vi "MasterAquisitionFile_FP.vi"() -> ()   [LabVIEW 2020]
uses:
  <vilib>/userDefined/High Color/IMAQdx.ctl
  <vilib>/vision/driver/IMAQdx.llb/IMAQdx Camera Control Mode.ctl
  <vilib>/vision/driver/IMAQdx.llb/IMAQdx Acquisition Mode.ctl
  <vilib>/vision/driver/IMAQdx.llb/IMAQdx Buffer Number Mode.ctl
  <vilib>/DAQmx/write.llb/DAQmx Write (Digital 1D Wfm NChan NSamp).vi
  <vilib>/DAQmx/read.llb/DAQmx Read (Digital 1D Bool 1Chan 1Samp).vi
  <vilib>/DAQmx/read.llb/DAQmx Read (Analog 1D Wfm NChan NSamp).vi
  <vilib>/Waveform/DWDTOps.llb/DWDT Digital to Boolean Array.vi
  <vilib>/DAQmx/create/channels.llb/DAQmx Create Channel (DO-Digital Output).vi
  <vilib>/DAQmx/configure/timing.llb/DAQmx Timing (Sample Clock).vi
  <vilib>/Waveform/DWDTOps.llb/DWDT Boolean Array to Digital.vi
  <vilib>/Waveform/DWDTOps.llb/DWDT Uncompress Digital.vi
  <vilib>/DAQmx/miscellaneous.llb/DAQmx Fill In Error Info.vi
  <vilib>/DAQmx/create/channels.llb/DAQmx Create Channel (DI-Digital Input).vi
  <vilib>/DAQmx/create/channels.llb/DAQmx Create Channel (AI-Voltage-Basic).vi
  <vilib>/DAQmx/configure/trigger.llb/DAQmx Start Trigger (Digital Edge).vi
  <vilib>/DAQmx/create/channels.llb/DAQmx Create Channel (CO-Pulse Generation-Frequency).vi
  <vilib>/DAQmx/configure/timing.llb/DAQmx Timing (Implicit).vi
  <vilib>/vision/driver/NI_Vision_Acquisition_Software.lvlib
  <resource>/objmgr/imaqdx.rc
  <resource>/objmgr/daqmx.rc
panel:
  in  "Analog Input Channels":tag="Dev2/ai0:3"
  out "Auditory":bool
  out "RPad":bool
  out "LPad":bool
  in  "Sol Stim Parameters":cluster{"Fs":dbl, "Samples":dbl}
  in  "LED Stim Parameters":cluster{"Fs":dbl, "Samples":dbl}
  in  "Generate Stimuli":bool=TRUE
  in  "Sol Duty Cycle (%)":dbl=50.0
  in  "Sol Freq":dbl=5.0
  in  "Sol Dur (s)":dbl=5.0
  in  "LED Duty Cycle (%)":dbl=10.0
  in  "LED Freq":dbl=10.0
  in  "LED Dur (s)":dbl=2.0
  out "Stimulus Order":digitalwaveform[](graph)=[{"t0"=timestamp(0 s since 1904-01-01), "dt"=5e-05, "Y"={"transitions"=[], "data"=array19221000x1[19221000 elements]}}, {"t0"=timestamp(0 s since 1904-01-01), "dt"=5e-05, "Y"={"transitions"=[], "data"=array19221000x1[19221000 elements]}}, {"t0"=timestamp(0 s since 1904-01-01), "dt"=5e-05, "Y"={"transitions"=[], "data"=array19221000x1[19221000 elements]}}]
  out "Solenoid Stim":digitalwaveform(graph)={"t0"=timestamp(0 s since 1904-01-01), "dt"=5e-05, "Y"={"transitions"=[], "data"=array100000x1[100000 elements]}}
  in  "Trial Offset (s)":dbl=45.0
  in  "Interstim (s)":dbl=45.0
  in  "Right Pad":dbl=1.0
  in  "Left Pad":dbl=1.0
  in  "Auditory":dbl=1.0
  in  "LED":dbl
  out "?":T1(plugin-control)
  in  "stop":bool
  out "?":T1(plugin-control)
  out "Behavior Cam Fs":dbl(knob) scale=0.0..200.0
  out "Behav Cam":bool
  out "Complete":bool
  out "Whisk Cam":bool
  out "Analog":bool
  out "MScan Trig":bool
  out "?":bool[](array[boolean])=[TRUE]
  out "Hexadecimal Data":u32=1 format="%x"
  out "Time Elapsed (Min)":cluster{dbl, dbl}(slide)={16.0, 0.0} scale=0.0..16.0 scale format="%#_2g"
  out "Whisker Camera":bool
  out "Analog Data":bool
  out "Analog Samples":i32=15417328
  in  "Device Analog Channel Labels":string[](array[string])=["forceSensor", "LPadSol", "RPadSol", "AudSol", "", "", "", ""]
  in  "?":cluster{"Analog Fs":u16}={"Analog Fs"=20000} {"Analog Fs" format="%0.0f"}
  in  "?":cluster{"WhiskerCam Fs":u16}={"WhiskerCam Fs"=150}
  out "Notes Size":i32=7
  out "Notes Reversed":string[](array[string])=["Experimenter", "Animal ID", "Isoflurane time", "Amplifier Gain", "Session ID", "Hemisphere", "Solenoid PSI"]
  out "Notes Array":string[](array[string])=["Solenoid PSI", "Hemisphere", "Session ID", "Amplifier Gain", "Isoflurane time", "Animal ID", "Experimenter"]
  in  "Notes:":T2={"Experimenter"="Kevin\n", "Animal ID"="Test", "Isoflurane time"="1145", "Amplifier Gain"="10000", "Session ID"="Imaging Session One", "Hemisphere"="RH", "Solenoid PSI"="10"}
  in  "Target Path":path=path "C:/Users/klt8/Documents" caption="Final Saved File Location"
  out "Dropped":u32(slide) caption="WhiskerCam" scale=0.0..150.0
  out "Current File Name":string="210517_13_39_46"
  in  "Time (min)":dbl(knob)=16.0 min=0.5 max=20.0 step=0.5 scale=0.0..20.0 scale format="%#_3g"
  in  "Temp Path":path=path "C:/Users/klt8/Documents/LabVIEW Temp Files" caption="Temporary File Path"
  out "Last Whisk Buffer":u32=115624
  out "Whisker Cam Fs":dbl(knob) scale=0.0..200.0 scale format="%#1_6g"
  # "Notes"
  # "Dropped Frames"
  # "LPAD"
  # "RPAD"
  # "AUD"
  # "Analog\nFs"
  # "Whisker\nFs"
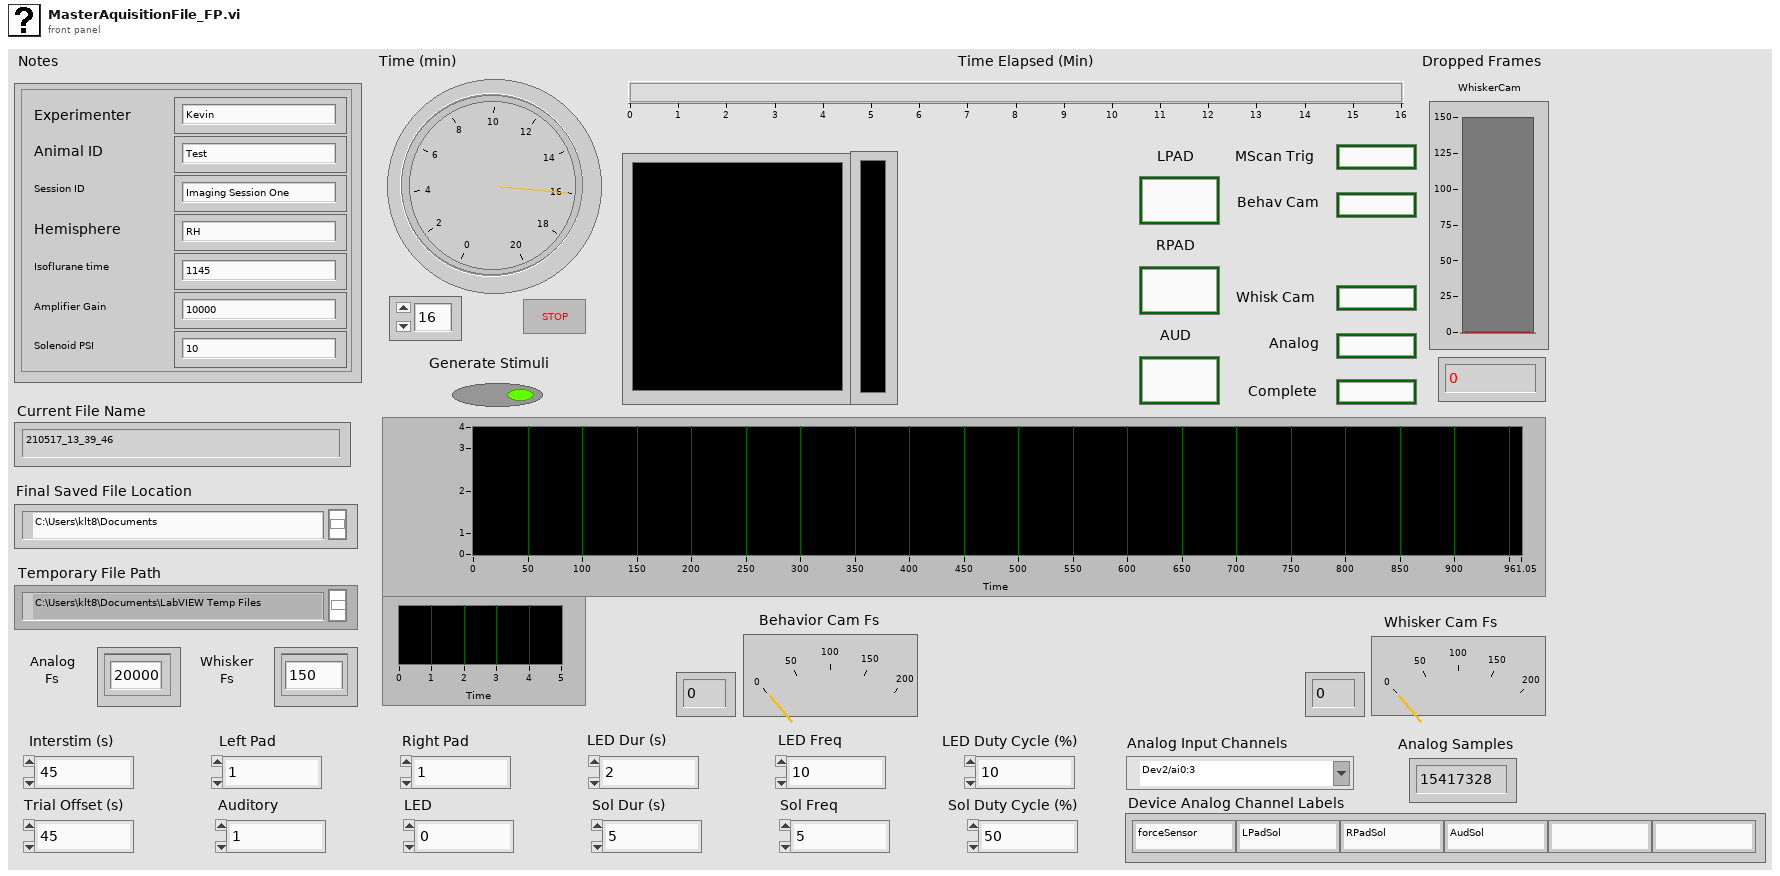
[diagram p1: front panel]
types:
  T1 = typedef "IMAQ Image.ctl" = refnum<image>
  T2 = cluster{"Experimenter":string, "Animal ID":string, "Isoflurane time":string, "Amplifier Gain":string, "Session ID":string, "Hemisphere":string, "Solenoid PSI":string}
  T3 = typedef "IMAQdx.ctl" = refnum<k21>
  T4 = enum16{"open", "open or create", "create or replace", "create", "open (read-only)"}
  T5 = typedef "NI_Vision_Acquisition_Software.lvlib/IMAQdx Camera Control Mode.ctl" = enum32{"Controller", "Listener"}
  T6 = enum16{"open", "replace", "create", "open or create", "replace or create", "replace or create with confirmation"}
  T7 = typedef "NI_Vision_Acquisition_Software.lvlib/IMAQdx Acquisition Mode.ctl" = enum32{"One Shot", "Continuous"}
  T8 = enum16{"big-endian, network order", "native, host order", "little-endian"}
  T9 = typedef "NI_Vision_Acquisition_Software.lvlib/IMAQdx Buffer Number Mode.ctl" = enum32{"Next", "Last", "Buffer Number", "Every", "Last New"}
  T10 = typedef "Image Type" = u32
  T11 = typedef "IMAQ AVI2 Refnum.ctl" = refnum<k20>
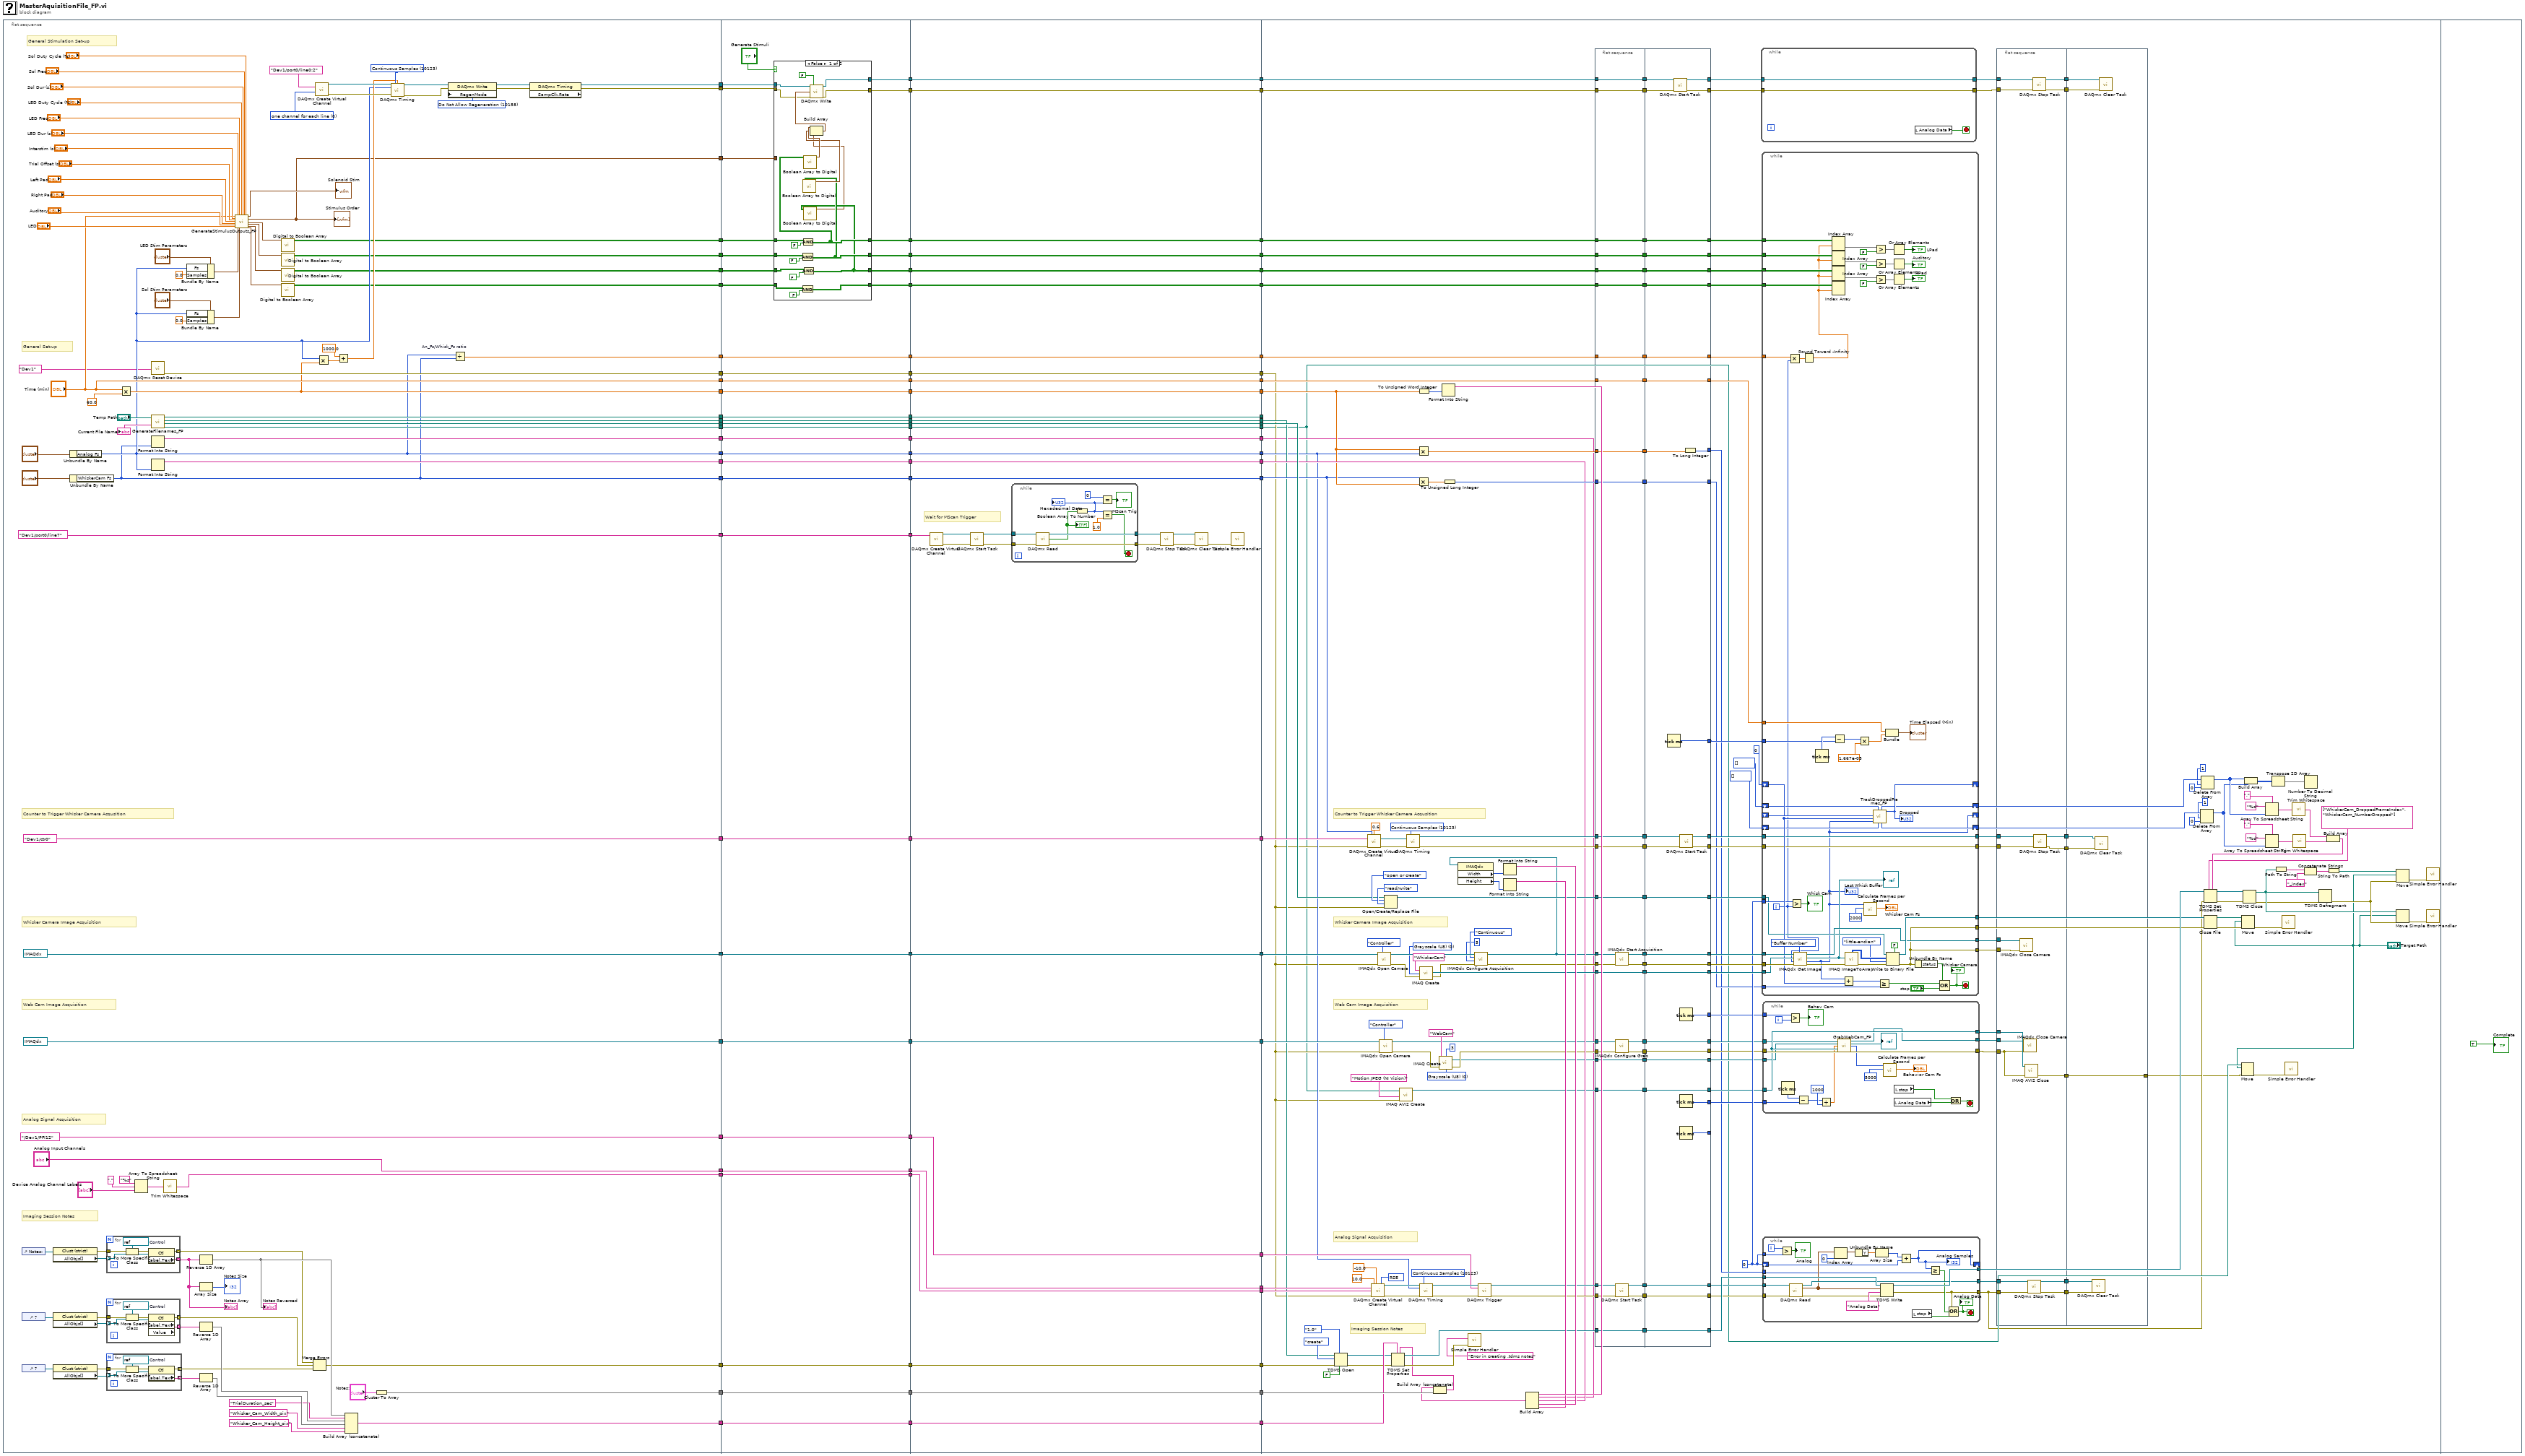
[diagram p0: block diagram]
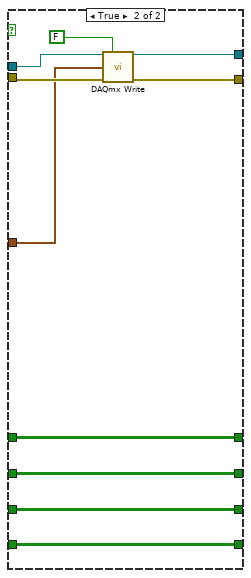
[diagram p2: hidden frame]
diagram:
  n1 = flat-sequence {
    tunnel: [tag "/Dev1/PFI12" ("Whisk Cam Trigger")] -> w57
    tunnel: [w105] -> w55
    tunnel: ["Time (min)"] -> w53
    tunnel: [w152] -> w51
    tunnel: [w151] -> w49
    tunnel: [w103] -> w47
    tunnel: [w102] -> w45
    tunnel: [w150] -> w43
    tunnel: [tag "Dev1/ctr0" ("Whisk Cam Counter")] -> w41
    tunnel: [w149] -> w39
    tunnel: ["Analog Input Channels"] -> w37
    tunnel: [T3 "cam2" ("Whisker Cam ID")] -> w35
    tunnel: [w148] -> w33
    tunnel: [w146] -> w31
    tunnel: [w147] -> w29
    tunnel: [T3 "cam1" ("WebCam ID")] -> w27
    tunnel: [tag "Dev1/port0/line7" ("MScan Trigger")] -> w25
    tunnel: [w143] -> w23
    tunnel: [w142] -> w21
    tunnel: [w141] -> w19
    tunnel: [w140] -> w17
    tunnel: [w101] -> w9
    tunnel: [w91] -> w7
    tunnel: [w90] -> w6
    tunnel: [w89] -> w5
    tunnel: [w88] -> w4
    tunnel: [w87] -> w3
    tunnel: [w86] -> w2
    tunnel: [w85] -> w1
    tunnel: w57 -> [w239]
    tunnel: [w239] -> w56
    tunnel: w55 -> [w238]
    tunnel: [w238] -> w54
    tunnel: w53 -> [w237]
    tunnel: [w237] -> w52
    tunnel: w51 -> [w236]
    tunnel: [w236] -> w50
    tunnel: w49 -> [w235]
    tunnel: [w235] -> w48
    tunnel: w47 -> [w234]
    tunnel: [w234] -> w46
    tunnel: w45 -> [w233]
    tunnel: [w233] -> w44
    tunnel: w43 -> [w232]
    tunnel: [w232] -> w42
    tunnel: w41 -> [w231]
    tunnel: [w231] -> w40
    tunnel: w39 -> [w230]
    tunnel: [w230] -> w38
    tunnel: w37 -> [w229]
    tunnel: [w229] -> w36
    tunnel: w35 -> [w228]
    tunnel: [w228] -> w34
    tunnel: w33 -> [w227]
    tunnel: [w227] -> w32
    tunnel: w31 -> [w226]
    tunnel: [w226] -> w30
    tunnel: w29 -> [w225]
    tunnel: [w225] -> w28
    tunnel: w27 -> [w224]
    tunnel: [w224] -> w26
    tunnel: w25 -> [w223]
    tunnel: [w223] -> w24
    tunnel: w23 -> [w222]
    tunnel: [w222] -> w22
    tunnel: w21 -> [w221]
    tunnel: [w221] -> w20
    tunnel: w19 -> [w220]
    tunnel: [w220] -> w18
    tunnel: w17 -> [w219]
    tunnel: [w219] -> w16
    tunnel: [w210] -> w15
    tunnel: [w209] -> w14
    tunnel: [w208] -> w13
    tunnel: [w207] -> w12
    tunnel: [w206] -> w11
    tunnel: [w205] -> w10
    tunnel: w9 -> [w218]
    tunnel: [w218] -> w8
    tunnel: w7 -> [w217]
    tunnel: w6 -> [w216]
    tunnel: w5 -> [w215]
    tunnel: w4 -> [w214]
    tunnel: w3 -> [w213]
    tunnel: w2 -> [w212]
    tunnel: w1 -> [w211]
    tunnel: [w284] -> w84
    tunnel: [w296] -> w83
    tunnel: [w297] -> w82
    tunnel: [w298] -> w81
    tunnel: [w299] -> w80
    tunnel: [w286] -> w79
    tunnel: [w300] -> w78
    tunnel: [w285] -> w77
    tunnel: [w301] -> w76
    tunnel: [w302] -> w75
    tunnel: [w303] -> w74
    tunnel: [w304] -> w73
    tunnel: [w305] -> w72
    tunnel: [w306] -> w71
    tunnel: [w307] -> w70
    tunnel: w56 -> [w307]
    tunnel: w54 -> [w306]
    tunnel: w52 -> [w305]
    tunnel: w50 -> [w304]
    tunnel: w48 -> [w303]
    tunnel: w46 -> [w302]
    tunnel: w44 -> [w301]
    tunnel: w42 -> [w285]
    tunnel: w40 -> [w300]
    tunnel: w38 -> [w286]
    tunnel: w36 -> [w299]
    tunnel: w34 -> [w298]
    tunnel: w32 -> [w297]
    tunnel: w30 -> [w296]
    tunnel: w28 -> [w284]
    tunnel: [w282] -> w69
    tunnel: w26 -> [w282]
    tunnel: w24 -> [w283]
    tunnel: w22 -> [w281]
    tunnel: [w281] -> w68
    tunnel: w20 -> [w280]
    tunnel: w18 -> [w279]
    tunnel: [w280] -> w67
    tunnel: [w279] -> w66
    tunnel: w16 -> [w278]
    tunnel: [w278] -> w65
    tunnel: [w277] -> w64
    tunnel: w15 -> [w277]
    tunnel: [w276] -> w63
    tunnel: w14 -> [w276]
    tunnel: [w275] -> w62
    tunnel: w13 -> [w275]
    tunnel: [w274] -> w61
    tunnel: w12 -> [w274]
    tunnel: [w273] -> w60
    tunnel: w11 -> [w273]
    tunnel: w10 -> [w272]
    tunnel: [w272] -> w59
    tunnel: [w271] -> w58
    tunnel: w8 -> [w271]
    tunnel: w84 -> [w406]
    tunnel: w83 -> [w415]
    tunnel: w82 -> [w360]
    tunnel: w81 -> [w414]
    tunnel: w80 -> [w413]
    tunnel: w79 -> [w412]
    tunnel: w78 -> [w411]
    tunnel: w77 -> [w410]
    tunnel: w76 -> [w379]
    tunnel: w75 -> [w369]
    tunnel: w74 -> [w409]
    tunnel: w73 -> [w368]
    tunnel: w72 -> [w403]
    tunnel: w71 -> [w408]
    tunnel: w70 -> [w407]
    tunnel: w69 -> [w394]
    tunnel: w68 -> [w359]
    tunnel: w67 -> [w375]
    tunnel: w66 -> [w373]
    tunnel: w65 -> [_]
    tunnel: w64 -> [w328]
    tunnel: w63 -> [w326]
    tunnel: w62 -> [w332]
    tunnel: w61 -> [w331]
    tunnel: w60 -> [w330]
    tunnel: w59 -> [w329]
    tunnel: w58 -> [w348]
    frame #0 {
      w120 = 10158 items=["Allow Regeneration"=10097, "Do Not Allow Regeneration"=10158] ("RegenMode")
      w121 = 10123 items=["Finite Samples"=10178, "Continuous Samples"=10123, "Hardware Timed Single Point"=12522] ("sample mode")
      w124 = 0 items=["one channel for each line", "one channel for all lines"] ("line grouping")
      # "General Stimulation Set-up"
      # "General Set-up"
      # "Whisker Camera Image Acquisition"
      # "Imaging Session Notes"
      # "Counter to Trigger Whisker Camera Acqusition"
      # "Web Cam Image Acquisition"
      # "Analog Signal Acquisition"
      n2 = control-ref of="Notes:"() -> (w168:refnum<vi>)
      n3 = control-ref of="?"() -> (w166:refnum<vi>)
      n4 = control-ref of="?"() -> (w159:refnum<vi>)
      n5 = property class="Clust (strict)"(reference=w168) -> (error out=w167:errorcluster, "AllObjs[]"=w169:refnum<vi>[])  [unwired: 1 in, 1 out]
      n6 = property class="Clust (strict)"(reference=w166) -> (error out=w164:errorcluster, "AllObjs[]"=w165:refnum<vi>[])  [unwired: 1 in, 1 out]
      n7 = property class="Clust (strict)"(reference=w159) -> (error out=w160:errorcluster, "AllObjs[]"=w162:refnum<vi>[])  [unwired: 1 in, 1 out]
      n8 = Unbundle By Name("?") -> ("Analog Fs"=w103:u16)
      n9 = Unbundle By Name("?") -> ("WhiskerCam Fs"=w102:u16)
      n10 = for {
        tunnel: [w187] -> w174 mode=indexing
        tunnel: w169 -> [w186] mode=indexing
        tunnel: w167 -> [w185]
        tunnel: [w183] -> w173 mode=indexing
        w188 = refnum<vi> refnum  # Control
        n11 = To More Specific Class(target class=w188, reference=w186, error in=w185) -> (specific class reference=w189:refnum<vi>, error out=w184:errorcluster)
        n12 = property class="Ctl"(reference=w189, error in=w184) -> (error out=w183:errorcluster, "Label.Text"=w187:string)  [unwired: 1 out]
      }
      "Notes Array" <- w174
      n13 = for {
        tunnel: [w194] -> w163 mode=indexing
        tunnel: w165 -> [w193] mode=indexing
        tunnel: w164 -> [w192]
        tunnel: [w190] -> w172 mode=indexing
        w195 = refnum<vi> refnum  # Control
        n14 = To More Specific Class(target class=w195, reference=w193, error in=w192) -> (specific class reference=w196:refnum<vi>, error out=w191:errorcluster)
        n15 = property class="Ctl" props=["Label", "Text", "Value"](reference=w196, error in=w191) -> (error out=w190:errorcluster, "Label.Text"=w194:string)  [unwired: 2 out]
      }
      n16 = for {
        tunnel: [w201] -> w161 mode=indexing
        tunnel: w162 -> [w200] mode=indexing
        tunnel: w160 -> [w199]
        tunnel: [w197] -> w171 mode=indexing
        w202 = refnum<vi> refnum  # Control
        n17 = To More Specific Class(target class=w202, reference=w200, error in=w199) -> (specific class reference=w203:refnum<vi>, error out=w198:errorcluster)
        n18 = property class="Ctl"(reference=w203, error in=w198) -> (error out=w197:errorcluster, "Label.Text"=w201:string)  [unwired: 1 out]
      }
      n19 = Multiply(x="Time (min)", y=60.0) -> (x*y=w105:dbl)
      n20 = Array To Spreadsheet String(delimiter (Tab)=",", array="Device Analog Channel Labels", 3:"%s" ("format string")) -> (spreadsheet string=w176:string)
      n21 = call <vilib>:"DAQmx Reset Device.vi"("device in"=tag "Dev1" ("NI Board")) -> ("error out"=w148:errorcluster)  [unwired: 14 in]
      n22 = call "GenerateFilenames_FP.vi"("path"="Temp Path") -> ("WebCam Path"=w143:path, "Basler Path"=w146:path, "TDMS Path"=w141:path, "MScan Path"=w140:path, "Analog file name"=→"Current File Name":string)  [unwired: 2 in]
      n23 = Format Into String(w102) -> (resulting string=w152:string)  [unwired: 3 in, 1 out]
      n24 = Format Into String(w103) -> (resulting string=w151:string)  [unwired: 3 in, 1 out]
      n25 = call <vilib>:"Trim Whitespace.vi"("string"=w176) -> ("trimmed string"=w149:string)  [unwired: 1 in]
      n26 = Bundle By Name(cluster="LED Stim Parameters", "Fs"=w103, "Samples"=0.0) -> (w110:cluster{"Fs":dbl, "Samples":dbl})
      n27 = Bundle By Name(cluster="Sol Stim Parameters", "Fs"=w103, "Samples"=0.0) -> (w109:cluster{"Fs":dbl, "Samples":dbl})
      n28 = Reverse 1D Array(array=w174) -> (reversed array=w175:string[])
      "Notes Reversed" <- w175
      n29 = Array Size(array=w174) -> (size(s)=→"Notes Size":i32)
      n30 = Reverse 1D Array(array=w163) -> (reversed array=w181:string[])
      n31 = Reverse 1D Array(array=w161) -> (reversed array=w182:string[])
      n32 = call "GenerateStimulusOutputs_FP.vi"("Trial duration (min)"="Time (min)", "Rest duration(s)"="Interstim (s)", "trial offset (s)"="Trial Offset (s)", "Left Pad"="Left Pad", "Right Pad"="Right Pad", "Auditory"="Auditory", "LED"="LED", "LED Stim Duration (s)"="LED Dur (s)", "LED Stim Parameters"=w110, "LED Frequency"="LED Freq", "Sol Stim Parameters"=w109, "LED duty cycle (%)"="LED Duty Cycle (%)", "Sol Stim Duration (s)"="Sol Dur (s)", "Sol Frequency"="Sol Freq", "Sol Duty Cycle (%)"="Sol Duty Cycle (%)") -> ("Solenoid Stim Waveforms"=→"Solenoid Stim":digitalwaveform, "Stimulus Digital Outputs"=w87:digitalwaveform[], "Left Pad Out"=w99:digitalwaveform, "Auditory Out"=w126:digitalwaveform, "Right Pad Out"=w125:digitalwaveform, "LED Out"=w104:digitalwaveform)  [unwired: 7 in]
      "Stimulus Order" <- w87
      n33 = call-poly <vilib>:"Digital to Boolean Array.vi"("digital waveform"=w99) -> ("boolean array"=w86:bool[][])  [unwired: 9 in, 1 out]
      n34 = call-poly <vilib>:"Digital to Boolean Array.vi"("digital waveform"=w126) -> ("boolean array"=w89:bool[][])  [unwired: 9 in, 1 out]
      n35 = call-poly <vilib>:"Digital to Boolean Array.vi"("digital waveform"=w125) -> ("boolean array"=w88:bool[][])  [unwired: 9 in, 1 out]
      n36 = call-poly <vilib>:"Digital to Boolean Array.vi"("digital waveform"=w104) -> ("boolean array"=w85:bool[][])  [unwired: 9 in, 1 out]
      n37 = Merge Errors(w173, w172, w171) -> (w142:errorcluster)
      n38 = call-poly <vilib>:"DAQmx Create Virtual Channel.vi"("lines"=tag "Dev1/port0/line0:2", "line grouping"=w124) -> ("task out"=w123:refnum<k21>, "error out"=w122:errorcluster)  [unwired: 12 in]
      n39 = Multiply(x=w103, y=w105) -> (x*y=w108:dbl)
      n40 = Add(x=1000.0, y=w108) -> (x+y=w106:dbl)
      n41 = Build Array (concatenate)(w175, "TrialDuration_sec", w181, w182, "Whisker_Cam_Width_pix", "Whisker_Cam_Height_pix") -> (w147:string[])
      n42 = Cluster To Array(cluster="Notes:") -> (array=w150:string[])
      n43 = call-poly <vilib>:"DAQmx Timing.vi"("task/channels in"=w123, "sample mode"=w121, "samples per channel"=w106, "rate"=w103, "error in"=w122) -> ("task out"=w117:refnum<k21>, "error out"=w116:errorcluster)  [unwired: 9 in]
      n44 = property class="DAQmx Write"(reference=w117, error in=w116, "RegenMode"=w120) -> (reference out=w118:refnum<k21>, error out=w119:errorcluster)
      n45 = Divide "An_Fs/Whisk_Fs ratio"(x=w103, y=w102) -> (x/y=w101:dbl)
      n46 = property class="DAQmx Timing" props=["SampClk.Rate"](reference=w118, error in=w119) -> (reference out=w91:refnum<k21>, error out=w90:errorcluster)  [unwired: 1 out]
    }
    frame #1 {
      n47 = case shown="False" "Generate Stimuli" {
        tunnel: w217 -> [w247 w270]
        tunnel: w216 -> [w246 w269]
        tunnel: [w244 w268] -> w210
        tunnel: [w245 w267] -> w209
        tunnel: w215 -> [w259 w266]
        tunnel: w214 -> [w260 w265]
        tunnel: [w243 w263] -> w208
        tunnel: [w242 w266] -> w207
        tunnel: [w241 w265] -> w206
        tunnel: [w253 w262] -> w205
        tunnel: w213 -> [_ w264]
        tunnel: w212 -> [w254 w263]
        tunnel: w211 -> [w252 w262]
        frame False {
          n48 = Compound Arithmetic op=AND(w259, FALSE) -> (w242:bool[][])
          n49 = call-poly <vilib>:"Boolean Array to Digital.vi"("boolean array"=w242) -> ("digital waveform"=w249:digitalwaveform)  [unwired: 9 in, 1 out]
          n50 = Compound Arithmetic op=AND(w252, FALSE) -> (w253:bool[][])
          n51 = Compound Arithmetic op=AND(w254, FALSE) -> (w243:bool[][])
          n52 = call-poly <vilib>:"Boolean Array to Digital.vi"("boolean array"=w243) -> ("digital waveform"=w250:digitalwaveform)  [unwired: 9 in, 1 out]
          n53 = Compound Arithmetic op=AND(w260, FALSE) -> (w241:bool[][])
          n54 = call-poly <vilib>:"Boolean Array to Digital.vi"("boolean array"=w241) -> ("digital waveform"=w240:digitalwaveform)  [unwired: 9 in, 1 out]
          n55 = Build Array(w250, w249, w240) -> (w248:digitalwaveform[])
          n56 = call-poly <vilib>:"DAQmx Write.vi"("task/channels in"=w247, "auto start"=FALSE, "data"=w248, "error in"=w246) -> ("task out"=w244:refnum<k21>, "error out"=w245:errorcluster)  [unwired: 9 in, 1 out]
        }
        frame True {
          n57 = call-poly <vilib>:"DAQmx Write.vi"("task/channels in"=w270, "auto start"=FALSE, "data"=w264, "error in"=w269) -> ("task out"=w268:refnum<k21>, "error out"=w267:errorcluster)  [unwired: 9 in, 1 out]
        }
      }
    }
    frame #2 {
      # "Wait for MScan Trigger"
      n58 = call-poly <vilib>:"DAQmx Create Virtual Channel.vi"("lines"=w283) -> ("task out"=w291:refnum<k21>, "error out"=w292:errorcluster)  [unwired: 13 in]
      n59 = call <vilib>:"DAQmx Start Task.vi"("task/channels in"=w291, "error in"=w292) -> ("task out"=w295:refnum<k21>, "error out"=w294:errorcluster)  [unwired: 12 in]
      n60 = while {
        tunnel: w295 -> [w317]
        tunnel: w294 -> [w316]
        tunnel: [w314] -> w289
        tunnel: [w315] -> w290
        stop <- w309 stop-if-true
        n61 = call-poly <vilib>:"DAQmx Read.vi"("task/channels in"=w317, "error in"=w316) -> ("task out"=w315:refnum<k21>, "data"=w313:bool[], "error out"=w314:errorcluster)  [unwired: 11 in]
        "?" <- w313
        n62 = Boolean Array To Number(Boolean array=w313) -> (number=w308:u32)
        "Hexadecimal Data" <- w308
        n63 = Equal?(x=w308, y=u32 0) -> (x = y?=→"MScan Trig":bool)
        n64 = Equal?(x=w308, y=1.0) -> (x = y?=w309:bool)
      }
      n65 = call <vilib>:"DAQmx Stop Task.vi"("task/channels in"=w290, "error in"=w289) -> ("task out"=w288:refnum<k21>, "error out"=w287:errorcluster)  [unwired: 12 in]
      n66 = call <vilib>:"DAQmx Clear Task.vi"("task in"=w288, "error in"=w287) -> ("error out"=w293:errorcluster)  [unwired: 13 in]
      n67 = call <vilib>:"Simple Error Handler.vi"("error in (no error)"=w293) -> ()  [unwired: 4 in, 5 out]
    }
    frame #3 {
      w398 = T10 0 items=["Grayscale (U8)", "Grayscale (I16)", "Grayscale (SGL)", "Complex (CSG)", "RGB (U32)", "HSL (U32)", "RGB (U64)", "Grayscale (U16)"] ("Image Type")
      w386 = u32 0 ("y")
      w424 = 10123 items=["Finite Samples"=10178, "Continuous Samples"=10123, "Hardware Timed Single Point"=12522] ("sample mode")
      w423 = 10083 items=["default"=-1, "RSE"=10083, "NRSE"=10078, "Differential"=10106, "Pseudodifferential"=12529] ("input terminal configuration")
      w425 = 10123 items=["Finite Samples"=10178, "Continuous Samples"=10123, "Hardware Timed Single Point"=12522] ("sample mode")
      w421 = T10 0 items=["Grayscale (U8)", "Grayscale (I16)", "Grayscale (SGL)", "Complex (CSG)", "RGB (U32)", "HSL (U32)", "RGB (U64)", "Grayscale (U16)"] ("Image Type")
      # "Whisker Camera Image Acquisition"
      # "Imaging Session Notes"
      # "Counter to Trigger Whisker Camera Acqusition"
      # "Web Cam Image Acquisition"
      # "Analog Signal Acquisition"
      n68 = TDMS Open(6:FALSE ("disable buffering? (T)"), 7:enum16{"1.0", "2.0"}."1.0" ("file format version (2.0)"), 8:w375, 10:T4."create" ("operation (0:open)"), 11:w373) -> (0:w372:errorcluster, 3:w371:refnum<k34>)  [unwired: 2 in]
      n69 = call-poly <vilib>:"DAQmx Create Virtual Channel.vi"("frequency"=w379, "duty cycle"=0.6, "counter"=w411, "error in"=w360) -> ("task out"=w448:refnum<k21>, "error out"=w449:errorcluster)  [unwired: 10 in]
      n70 = call-poly <vilib>:"DAQmx Create Virtual Channel.vi"("maximum value"=10.0, "minimum value"=-10.0, "input terminal configuration"=w423, "physical channels"=w413, "name to assign"=w412, "error in"=w360) -> ("task out"=w457:refnum<k21>, "error out"=w458:errorcluster)  [unwired: 8 in]
      n71 = call <vilib>:"IMAQdx Open Camera.vi"("Camera Control Mode"=IMAQdx_Camera_Control_Mode."Controller", "error in"=w360, "Session In"=w414) -> ("error out"=w446:errorcluster, "Session Out"=w445:T3)  [unwired: 7 in]
      n72 = call <vilib>:"IMAQdx Open Camera.vi"("Camera Control Mode"=IMAQdx_Camera_Control_Mode."Controller", "error in"=w360, "Session In"=w394) -> ("error out"=w395:errorcluster, "Session Out"=w393:T3)  [unwired: 7 in]
      n73 = Open/Create/Replace File(file path (use dialog)=w415, error in=w360, operation (0:open)=T6."open or create", access (0:read/write)=enum16{"read/write", "read-only", "write-only"}."read/write") -> (refnum out=w456:refnum<file>)  [unwired: 2 in, 2 out]
      n74 = call "IMAQ AVI2 Create"("error in (no error)"=w360, "Codec"="Motion JPEG (NI Vision)", "AVI Path"=w359) -> ("AVI Refnum"=w381:T11)  [unwired: 7 in, 1 out]
      n75 = call-poly <vilib>:"DAQmx Timing.vi"("task/channels in"=w448, "sample mode"=w425, "error in"=w449) -> ("task out"=w466:refnum<k21>, "error out"=w467:errorcluster)  [unwired: 11 in]
      n76 = Multiply(x=w408, y=w369) -> (x*y=w493:dbl)
      n77 = Multiply(x=w379, y=w408) -> (x*y=w494:dbl)
      n78 = To Unsigned Word Integer(number=w408) -> (unsigned 16bit integer=w481:u16)
      n79 = call "IMAQ Create"("Image Name"="WhiskerCam", "Image Type"=w421, "error in (no error)"=w446) -> ("New Image"=w484:T1, "error out"=w447:errorcluster)  [unwired: 2 in]
      n80 = call-poly <vilib>:"DAQmx Timing.vi"("task/channels in"=w457, "sample mode"=w424, "rate"=w369, "error in"=w458) -> ("task out"=w459:refnum<k21>, "error out"=w460:errorcluster)  [unwired: 10 in]
      n81 = call "IMAQ Create"("Border Size"=3, "Image Name"="WebCam", "Image Type"=w398, "error in (no error)"=w395) -> ("New Image"=w391:T1, "error out"=w392:errorcluster)  [unwired: 1 in]
      n82 = Format Into String(w481) -> (resulting string=w502:string)  [unwired: 3 in, 1 out]
      n83 = To Unsigned Long Integer(number=w494) -> (unsigned 32bit integer=w495:u32)
      n84 = call <vilib>:"IMAQdx Configure Acquisition.vi"("error in"=w447, "Number of Buffers"=u32 5, "Continuous?"=IMAQdx_Acquisition_Mode."Continuous", "Session In"=w445) -> ("error out"=w451:errorcluster, "Session Out"=w370:T3)  [unwired: 6 in]
      n85 = property class="IMAQdx"(reference=w370) -> ("Width"=w482:u32, "Height"=w483:u32)  [unwired: 1 in, 2 out]
      n86 = call-poly <vilib>:"DAQmx Trigger.vi"("task/channels in"=w459, "source"=w407, "error in"=w460) -> ("task out"=w461:refnum<k21>, "error out"=w462:errorcluster)  [unwired: 11 in]
      n87 = Format Into String(w482) -> (resulting string=w501:string)  [unwired: 3 in, 1 out]
      n88 = Format Into String(w483) -> (resulting string=w500:string)  [unwired: 3 in, 1 out]
      n89 = Build Array(w502, w368, w409, w501, w500) -> (w366:string[])
      n90 = Build Array (concatenate)(w410, w366) -> (w416:string[])
      n91 = TDMS Set Properties(5:w416, 7:w406, 8:w372, 11:w371) -> (0:w480:errorcluster, 3:w479:refnum<k34>)  [unwired: 2 in, 2 out]
      n92 = call <vilib>:"Simple Error Handler.vi"("error source (\" \")"="Error in creating .tdms notes" ("error source (\" \")"), "error in (no error)"=w480) -> ()  [unwired: 3 in, 5 out]
      n93 = flat-sequence {
        tunnel: w370 -> [w613]
        tunnel: w451 -> [w612]
        tunnel: [w611] -> w513
        tunnel: [w610] -> w512
        tunnel: [w609] -> w511
        tunnel: w484 -> [w609]
        tunnel: [w608] -> w510
        tunnel: w456 -> [w608]
        tunnel: w461 -> [w607]
        tunnel: w462 -> [w606]
        tunnel: [w605] -> w509
        tunnel: [w604] -> w508
        tunnel: [w603] -> w507
        tunnel: w479 -> [w603]
        tunnel: w466 -> [w602]
        tunnel: [w602] -> w506
        tunnel: w467 -> [w601]
        tunnel: [w601] -> w505
        tunnel: w493 -> [w600]
        tunnel: [w600] -> w504
        tunnel: w495 -> [w599]
        tunnel: [w599] -> w503
        tunnel: w403 -> [w598]
        tunnel: [w598] -> w402
        tunnel: w393 -> [w597]
        tunnel: w392 -> [w596]
        tunnel: w391 -> [w595]
        tunnel: [w595] -> w390
        tunnel: [w594] -> w389
        tunnel: [w593] -> w388
        tunnel: [w592] -> w382
        tunnel: w381 -> [w592]
        tunnel: [w591] -> w357
        tunnel: w332 -> [w591]
        tunnel: [w590] -> w356
        tunnel: w331 -> [w590]
        tunnel: [w589] -> w355
        tunnel: w330 -> [w589]
        tunnel: [w588] -> w354
        tunnel: w329 -> [w588]
        tunnel: [w587] -> w349
        tunnel: w348 -> [w587]
        tunnel: w328 -> [w585]
        tunnel: [w586] -> w327
        tunnel: w326 -> [w586]
        tunnel: [w585] -> w325
        tunnel: [w638] -> w404
        tunnel: [w637] -> w405
        tunnel: [w645] -> w452
        tunnel: w513 -> [w645]
        tunnel: [w644] -> w453
        tunnel: w512 -> [w644]
        tunnel: [w643] -> w454
        tunnel: w511 -> [w643]
        tunnel: [w642] -> w455
        tunnel: w510 -> [w642]
        tunnel: [w641] -> w464
        tunnel: w509 -> [w641]
        tunnel: [w640] -> w463
        tunnel: w508 -> [w640]
        tunnel: [w639] -> w465
        tunnel: w507 -> [w639]
        tunnel: w506 -> [w634]
        tunnel: w505 -> [w636]
        tunnel: w504 -> [w625]
        tunnel: w503 -> [w635]
        tunnel: [w635] -> w365
        tunnel: [w633] -> w444
        tunnel: w402 -> [w632]
        tunnel: [w632] -> w401
        tunnel: [w631] -> w385
        tunnel: w390 -> [w631]
        tunnel: [w630] -> w383
        tunnel: w389 -> [w630]
        tunnel: [w629] -> w384
        tunnel: w388 -> [w629]
        tunnel: [w628] -> w378
        tunnel: w382 -> [w627]
        tunnel: [w627] -> w380
        tunnel: [w626] -> w377
        tunnel: [w624] -> w364
        tunnel: [w623] -> _
        tunnel: w357 -> [w622]
        tunnel: [w622] -> w353
        tunnel: [w621] -> w352
        tunnel: w356 -> [w621]
        tunnel: w355 -> [w620]
        tunnel: [w620] -> w351
        tunnel: w354 -> [w619]
        tunnel: [w619] -> w350
        tunnel: [w618] -> w347
        tunnel: w349 -> [w618]
        tunnel: [w617] -> w346
        tunnel: [w616] -> w345
        tunnel: w327 -> [w615]
        tunnel: w325 -> [w614]
        frame #0 {
          n94 = call <vilib>:"IMAQdx Start Acquisition.vi"("error in"=w612, "Session In"=w613) -> ("error out"=w610:errorcluster, "Session Out"=w611:T3)  [unwired: 8 in]
          n95 = call <vilib>:"IMAQdx Configure Grab.vi"("error in"=w596, "Session In"=w597) -> ("error out"=w593:errorcluster, "Session Out"=w594:T3)  [unwired: 8 in]
          n96 = call <vilib>:"DAQmx Start Task.vi"("task/channels in"=w607, "error in"=w606) -> ("task out"=w605:refnum<k21>, "error out"=w604:errorcluster)  [unwired: 12 in]
        }
        frame #1 {
          n97 = Tick Count (ms)() -> (millisecond timer value=w633:u32)
          n98 = call <vilib>:"DAQmx Start Task.vi"("task/channels in"=w614, "error in"=w615) -> ("task out"=w617:refnum<k21>, "error out"=w616:errorcluster)  [unwired: 12 in]
          n99 = Tick Count (ms)() -> (millisecond timer value=w628:u32)
          n100 = Tick Count (ms)() -> (millisecond timer value=w626:u32)
          n101 = Tick Count (ms)() -> (millisecond timer value=w623:u32)
          n102 = call <vilib>:"DAQmx Start Task.vi"("task/channels in"=w634, "error in"=w636) -> ("task out"=w638:refnum<k21>, "error out"=w637:errorcluster)  [unwired: 12 in]
          n103 = To Long Integer(number=w625) -> (32bit integer=w624:i32)
        }
      }
      n104 = while {
        tunnel: w346 -> [w541]
        tunnel: [w539] -> w341
        tunnel: w345 -> [w539]
        tunnel: [w541] -> w342
        stop <- w540 stop-if-true
        n105 = local read "Analog Data"() -> (w540:bool)
      }
      n106 = while {
        tunnel: [w691] -> w323
        tunnel: [w675] -> w478
        tunnel: [w699] -> w450
        tunnel: w452 -> [w698]
        tunnel: w453 -> [w697]
        tunnel: w454 -> [w696]
        tunnel: w455 -> [w669]
        shift-right: [w649] -> _
        shift-left: _ -> [w695]
        shift-right: [w694] -> _
        shift-left: u32 0 ("New Lost") -> [w690]
        shift-right: [w693] -> w492
        shift-left: u32[] [] ("NewBuffNum") -> [w648]
        shift-right: [w692] -> w468
        shift-left: u32[] [] ("NewNumLost") -> [w684]
        tunnel: w365 -> [w688]
        tunnel: w444 -> [w679]
        tunnel: w401 -> [w677]
        tunnel: [w675] -> w324
        tunnel: w386 -> [w674]
        tunnel: w405 -> [w672]
        tunnel: w404 -> [w671]
        tunnel: [w672] -> w339
        tunnel: [w671] -> w340
        tunnel: w353 -> [w655]
        tunnel: w352 -> [w654]
        tunnel: w351 -> [w653]
        tunnel: w350 -> [w652]
        tunnel: w347 -> [w650]
        i -> [w646]
        stop <- w685 stop-if-true
        n107 = Multiply(x=w650, y=w646) -> (x*y=w651:dbl)
        n108 = Greater?(x=w646, y=w674) -> (0:→"Whisk Cam":bool)
        n109 = call <vilib>:"IMAQdx Get Image.vi"("Buffer Number Mode (Next)"=IMAQdx_Buffer_Number_Mode."Buffer Number", "error in"=w697, "Buffer Number In"=w646, "Image In"=w696, "Session In"=w698) -> ("error out"=w705:errorcluster, "Buffer Number Out"=w649:u32, "Image Out"=w668:T1, "Session Out"=w691:T3)  [unwired: 3 in]
        "Last Whisk Buffer" <- w649
        "?" <- w668
        n110 = Round Toward -Infinity(1:w651) -> (0:w647:dbl)
        n111 = Tick Count (ms)() -> (millisecond timer value=w680:u32)
        n112 = Index Array(array=w655, index (row)=w647) -> (element=w661:bool[])  [unwired: 1 in]
        n113 = Index Array(array=w654, index (row)=w647) -> (element=w659:bool[])  [unwired: 1 in]
        n114 = Index Array(array=w653, index (row)=w647) -> (element=w657:bool[])  [unwired: 1 in]
        n115 = Index Array(array=w652, index (row)=w647) -> ()  [unwired: 1 in, 1 out]
        n116 = Subtract(x=w680, y=w679) -> (x-y=w683:u32)
        n117 = Add(x=w649, y=w690) -> (x+y=w689:u32)
        n118 = call "IMAQ ImageToArray"("error in (no error)"=w705, "Image"=w668) -> ("error out"=w704:errorcluster, "Image Pixels (U8)"=w703:u8[][])  [unwired: 2 in, 3 out]
        n119 = Multiply(x=w683, y=1.667e-05) -> (x*y=w682:dbl)
        n120 = call <vilib>:"Calculate Frames per Second.vi"("Update Interval (ms)"=u32 2000, "Buffer Number"=w649) -> ("Processed Frames/s"=→"Whisker Cam Fs":dbl)  [unwired: 7 in, 2 out]
        n121 = call "TrackDroppedFrames_FP.vi"("NumLost"=w684, "BuffNum"=w648, "Curr Buffer"=w649, "Prev Lost"=w690, "Prev Buffer"=w695) -> ("New Lost"=w694:u32, "NewNumLost"=w692:u32[], "NewBuffNum"=w693:u32[])  [unwired: 4 in]
        "Dropped" <- w694
        n122 = Greater?(x=w661, y=FALSE ("Boolean")) -> (0:w660:bool[])
        n123 = Greater?(x=w659, y=FALSE ("Boolean")) -> (0:w658:bool[])
        n124 = Greater?(x=w657, y=FALSE ("Boolean")) -> (0:w656:bool[])
        n125 = Greater Or Equal?(x=w689, y=w688) -> (x >= y?=w686:bool)
        n126 = Bundle("Time (min)"=w677, w682) -> (→"Time Elapsed (Min)":cluster{"Time (min)":dbl, dbl})  [unwired: 1 in]
        n127 = Write to Binary File(file (use dialog)=w669, data=w703, error in=w704, 5:FALSE ("prepend array or string size? (T)"), 9:T8."little-endian" ("byte order (0:big-endian, network order)")) -> (refnum out=w699:refnum<file>, error out=w675:errorcluster)  [unwired: 1 in, 1 out]
        n128 = Or Array Elements(Boolean array=w660) -> (logical OR=→"LPad":bool)
        n129 = Or Array Elements(Boolean array=w658) -> (logical OR=→"Auditory":bool)
        n130 = Or Array Elements(Boolean array=w656) -> (logical OR=→"RPad":bool)
        n131 = Unbundle By Name(w675) -> ("status"=w687:bool)
        n132 = Compound Arithmetic op=OR(w687, w686, "stop") -> (w685:bool)
        "Whisker Camera" <- w685
      }
      n133 = while {
        tunnel: w463 -> [w584]
        tunnel: w464 -> [w583]
        tunnel: w465 -> [w582]
        tunnel: [w581] -> w485
        tunnel: [w569] -> w333
        tunnel: [w580] -> w334
        shift-right: [w573] -> _
        shift-left: w386 -> [w574]
        tunnel: w386 -> [w565]
        tunnel: w364 -> [w563]
        i -> [w566]
        stop <- w570 stop-if-true
        n134 = Greater?(x=w566, y=w565) -> (0:→"Analog":bool)
        n135 = call-poly <vilib>:"DAQmx Read.vi"("task/channels in"=w583, "error in"=w584) -> ("task out"=w580:refnum<k21>, "data"=w578:waveform(dbl)[], "error out"=w572:errorcluster)  [unwired: 11 in]
        n136 = Index Array(array=w578, index=0) -> (element=w576:waveform(dbl))
        n137 = Unbundle By Name(w576) -> ("Y"=w575:dbl[])
        n138 = Array Size(array=w575) -> (size(s)=w568:i32)
        n139 = TDMS Write(0:w582, 5:"Analog Data" ("group name in (Untitled)"), 9:w578, 11:w572) -> (4:w581:refnum<k34>, 15:w569:errorcluster)  [unwired: 2 in, 2 out]
        n140 = Add(x=w568, y=w574) -> (x+y=w573:u32)
        "Analog Samples" <- w573
        n141 = local read "stop"() -> (w564:bool)
        n142 = Greater Or Equal?(x=w573, y=w563) -> (x >= y?=w571:bool)
        n143 = Compound Arithmetic op=OR(w564, w569, w571) -> (w570:bool)
        "Analog Data" <- w570
      }
      n144 = while {
        tunnel: w385 -> [w549]
        tunnel: w383 -> [w548]
        tunnel: w384 -> [w552]
        tunnel: w380 -> [w551]
        tunnel: [w542] -> w320
        tunnel: [w553] -> w322
        tunnel: [w551] -> w321
        tunnel: w378 -> [w555]
        tunnel: w377 -> [w554]
        i -> [w556]
        stop <- w544 stop-if-true
        n145 = Tick Count (ms)() -> (millisecond timer value=w560:u32)
        n146 = Greater?(x=w555, y=w556) -> (0:→"Behav Cam":bool)
        n147 = Subtract(x=w560, y=w554) -> (x-y=w561:u32)
        n148 = Divide(x=w561, y=u32 1000) -> (x/y=w550:dbl)
        n149 = call "GrabWebCam_FP.vi"("Session In"=w548, "Image In"=w549, "Trial Time"=w550, "AVI Refnum"=w551, "error in"=w552) -> ("Session Out"=w542:T3, "WebCam Img Out"=→"?":T1, "Buffer Number Out"=w546:u32, "error out"=w553:errorcluster)  [unwired: 7 in]
        n150 = call <vilib>:"Calculate Frames per Second.vi"("Update Interval (ms)"=u32 5000, "Buffer Number"=w546) -> ("Processed Frames/s"=→"Behavior Cam Fs":dbl)  [unwired: 7 in, 2 out]
        n151 = local read "Analog Data"() -> (w545:bool)
        n152 = local read "stop"() -> (w543:bool)
        n153 = Compound Arithmetic op=OR(w543, w545) -> (w544:bool)
      }
      n154 = flat-sequence {
        tunnel: [w531] -> w344
        tunnel: [w530] -> w343
        tunnel: w342 -> [w520]
        tunnel: w341 -> [w529]
        tunnel: w340 -> [w528]
        tunnel: w339 -> [w527]
        tunnel: [w526] -> w338
        tunnel: [w525] -> w337
        tunnel: [w524] -> w336
        tunnel: [w523] -> w335
        tunnel: w334 -> [w522]
        tunnel: w333 -> [w521]
        tunnel: w324 -> [w519]
        tunnel: w323 -> [w518]
        tunnel: w322 -> [w516]
        tunnel: w321 -> [w517]
        tunnel: w320 -> [w515]
        tunnel: [w514] -> w319
        tunnel: w344 -> [w538]
        tunnel: w343 -> [w537]
        tunnel: w338 -> [w536]
        tunnel: w337 -> [w535]
        tunnel: w336 -> [w534]
        tunnel: w335 -> [w533]
        tunnel: w319 -> [w532]
        tunnel: [w532] -> w318
        frame #0 {
          n155 = call <vilib>:"IMAQdx Close Camera.vi"("error in"=w519, "Session In"=w518) -> ()  [unwired: 9 in, 1 out]
          n156 = call <vilib>:"IMAQdx Close Camera.vi"("error in"=w516, "Session In"=w515) -> ()  [unwired: 9 in, 1 out]
          n157 = call "IMAQ AVI2 Close"("error in (no error)"=w516, "AVI Refnum"=w517) -> ("error out"=w514:errorcluster)  [unwired: 9 in]
          n158 = call <vilib>:"DAQmx Stop Task.vi"("task/channels in"=w522, "error in"=w521) -> ("task out"=w524:refnum<k21>, "error out"=w523:errorcluster)  [unwired: 12 in]
          n159 = call <vilib>:"DAQmx Stop Task.vi"("task/channels in"=w520, "error in"=w529) -> ("task out"=w531:refnum<k21>, "error out"=w530:errorcluster)  [unwired: 12 in]
          n160 = call <vilib>:"DAQmx Stop Task.vi"("task/channels in"=w528, "error in"=w527) -> ("task out"=w525:refnum<k21>, "error out"=w526:errorcluster)  [unwired: 12 in]
        }
        frame #1 {
          n161 = call <vilib>:"DAQmx Clear Task.vi"("task in"=w534, "error in"=w533) -> ()  [unwired: 13 in, 1 out]
          n162 = call <vilib>:"DAQmx Clear Task.vi"("task in"=w535, "error in"=w536) -> ()  [unwired: 13 in, 1 out]
          n163 = call <vilib>:"DAQmx Clear Task.vi"("task in"=w538, "error in"=w537) -> ()  [unwired: 13 in, 1 out]
        }
      }
      n164 = Delete From Array(array=w468, length=1, index=0) -> (array with subset deleted=w498:u32[])  [unwired: 1 out]
      n165 = Delete From Array(array=w492, length=1, index=0) -> (array with subset deleted=w499:u32[])  [unwired: 1 out]
      n166 = Close File(refnum=w450, error in=w478) -> (path=w470:path, error out=w471:errorcluster)
      n167 = Move(source path=w359, error in=w318, 10:"Target Path") -> (error out=w387:errorcluster)  [unwired: 2 in, 2 out]
      n168 = Move(source path=w470, error in=w471, 10:"Target Path") -> (error out=w473:errorcluster)  [unwired: 2 in, 2 out]
      n169 = Build Array(w499, w498) -> (w496:u32[][])
      n170 = Array To Spreadsheet String(delimiter (Tab)=",", array=w499, 3:"%d" ("format string")) -> (spreadsheet string=w488:string)
      n171 = Array To Spreadsheet String(delimiter (Tab)=",", array=w498, 3:"%d" ("format string")) -> (spreadsheet string=w489:string)
      n172 = Transpose 2D Array(2D array=w496) -> (transposed array=w497:u32[][])
      n173 = call <vilib>:"Simple Error Handler.vi"("error in (no error)"=w473) -> ()  [unwired: 1 in, 8 out]
      n174 = call <vilib>:"Simple Error Handler.vi"("error in (no error)"=w387) -> ()  [unwired: 1 in, 8 out]
      n175 = call <vilib>:"Trim Whitespace.vi"("string"=w488) -> ("trimmed string"=w363:string)  [unwired: 1 in]
      n176 = call <vilib>:"Trim Whitespace.vi"("string"=w489) -> ("trimmed string"=w490:string)  [unwired: 1 in]
      n177 = Number To Decimal String(number=w497) -> ()  [unwired: 1 in, 1 out]
      n178 = Build Array(w363, w490) -> (w491:string[])
      n179 = TDMS Set Properties(5:w491, 7:string[] ["WhiskerCam_DroppedFrameIndex", "WhiskerCam_NumberDropped"] ("channel name(s) in (Untitled)"), 8:w333, 11:w485) -> (0:w486:errorcluster, 3:w487:refnum<k34>)  [unwired: 2 in, 2 out]
      n180 = TDMS Close(8:w486, 11:w487) -> (0:w469:errorcluster, 3:w474:path)
      n181 = Path To String(path=w474) -> (string=w362:string)
      n182 = Concatenate Strings(w362, "_index" ("string")) -> (w475:string)
      n183 = TDMS Defragment(4:w469, 7:w474) -> (0:w477:errorcluster)
      n184 = String To Path(string=w475) -> (path=w476:path)
      n185 = Move(source path=w474, error in=w477, 10:"Target Path") -> (error out=w472:errorcluster)  [unwired: 2 in, 2 out]
      n186 = Move(source path=w476, error in=w477, 10:"Target Path") -> (error out=w361:errorcluster)  [unwired: 2 in, 2 out]
      n187 = call <vilib>:"Simple Error Handler.vi"("error in (no error)"=w361) -> ()  [unwired: 1 in, 8 out]
      n188 = call <vilib>:"Simple Error Handler.vi"("error in (no error)"=w472) -> ()  [unwired: 1 in, 8 out]
    }
    frame #4 {
      "Complete" <- TRUE ("Data Acquisition - Complete")
    }
  }
